vi "F020_dout_set.vi"(8 "error in":errorcluster, 10 "Cluster":T1={"ADDRESS"=170, "DOUT CHANNEL"=0, "DOUT value"=1, "DOUT timeout[sec]"=0} {"DOUT timeout[sec]" format="%04x"; "DOUT value" format="%.0x"; "ADDRESS" format="%.0x"}, 11 "COM in":string="}") -> (0 "error out":errorcluster, 3 "COM out":string="}")   [LabVIEW 2016]
doc: "This example performs a serial port write and a serial port read. The parameters set for the serial port must match the parameters of the connected instrument or device. The VISA Configure Serial Port VI sets the configuration parameters. The front panel displays the controls used to configure the basic parameters, such as baud rate, data bits, and parity. The VI passes the VISA resource name to other VIs that perform operations on that VISA resource. The VISA Write function sends a command to the serial device and the VISA Read function returns data based on the command. The VISA Close function then closes the reference to the serial device. It is important to close the reference; otherwise, further communication through that port might not be possible."
panel:
  # "loopback: <xxAABB>\nwr_dout:   <xxAA11aabbccdd> aa=ch, bb=val, ccdd=timeout[sec]"
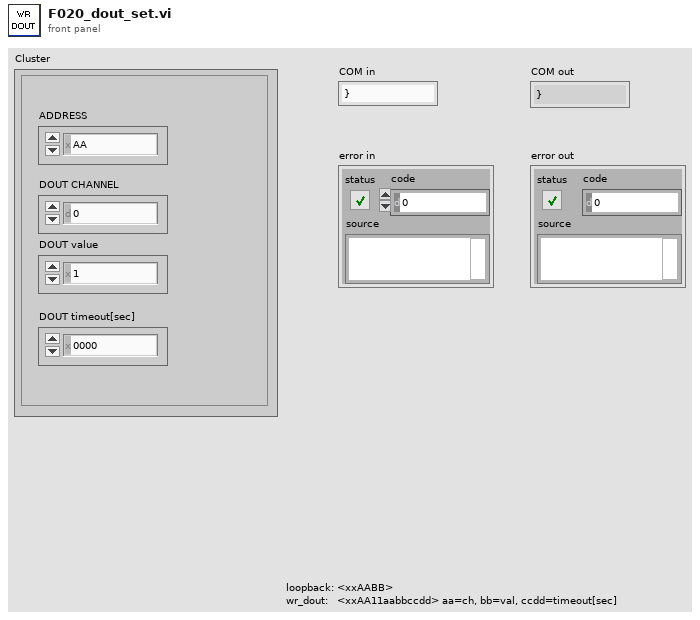
[diagram p1: front panel]
types:
  T1 = cluster{"ADDRESS":u8, "DOUT CHANNEL":u8, "DOUT value":u8, "DOUT timeout[sec]":u16}
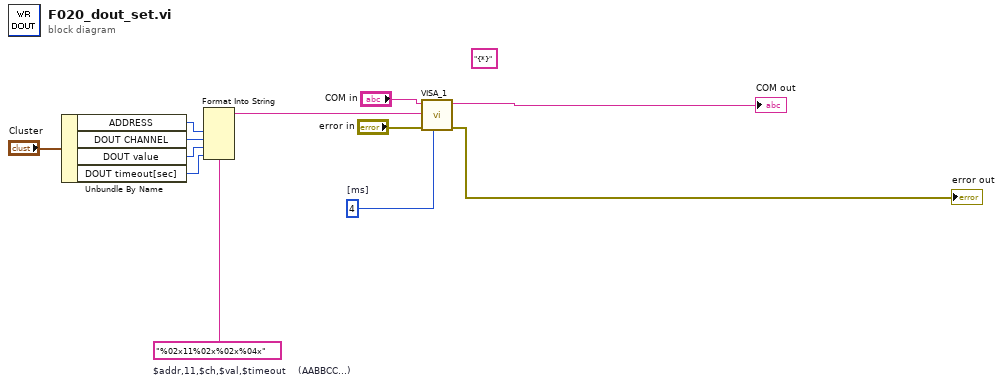
[diagram p0: block diagram]
diagram:
  w3 = u32 4  # [ms]
  (unwired) "{*}" ("regular expression")
  w9 = "%02x11%02x%02x%04x"  # $addr,11,$ch,$val,$timeout    (AABBCC...)
  n1 = Unbundle By Name("Cluster") -> ("ADDRESS"=w4:u8, "DOUT CHANNEL"=w7:u8, "DOUT value"=w6:u8, "DOUT timeout[sec]"=w5:u16)
  n2 = Format Into String(format string=w9, w4, w7, w6, w5) -> (resulting string=w1:string)  [unwired: 2 in, 1 out]
  n3 = call "VISA_1.vi"("delay[ms]"=w3, "error in"="error in", "wr_buf"=w1, "COM in"="COM in") -> ("error out"=→"error out":errorcluster, "COM out"=→"COM out":string)  [unwired: 4 in, 2 out]
